vi "Get Differential Pressure Release Valve Test Settings.vi"(11 "Model in":refnum<class "Model.lvclass">) -> (2 "Differential Pressure Release Valve Test Settings":T1 {"Sample Time (s)" format="%.4f"; "Process Time (s)" format="%.4f"; "Max Moment (NM)" format="%.4f"; "Max Over Force (N)" format="%.4f"}, 3 "Model out":refnum<class "Model.lvclass">)   [LabVIEW 2016]
uses:
  Model.lvclass
  Typedefs/DifferentialPressureReleaseValveTestSettings.ctl
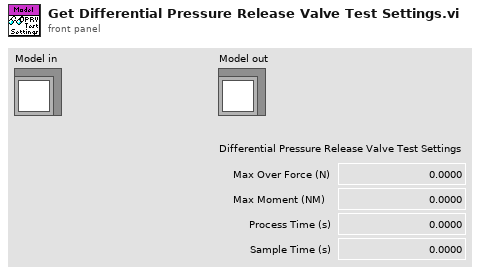
[diagram p1: front panel]
types:
  T1 = typedef "DifferentialPressureReleaseValveTestSettings.ctl" = cluster{"Max Over Force (N)":dbl, "Max Moment (NM)":dbl, "Process Time (s)":dbl, "Sample Time (s)":dbl}
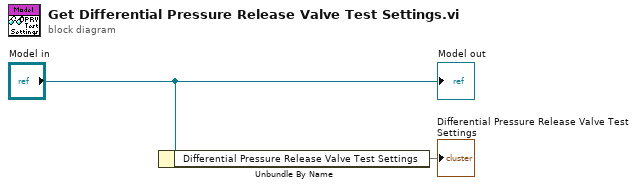
[diagram p0: block diagram]
diagram:
  n1 = Unbundle By Name("Model in") -> ("Differential Pressure Release Valve Test Settings"=→"Differential Pressure Release Valve Test Settings")
  "Model out" <- "Model in"
